vi "Z_state.vi"(9 "Alarm":bool[](array[boolean])=[FALSE, FALSE], 10 "Z_In":T4={"Z_Source"=enum."hand", "Z_Set_State"=enum."initialization", "ZM_State"=enum."initialization"}, 11 "Z_state in":refnum<class "valve_VCH_Z_state.lvclass">) -> (3 "Z_state out":refnum<class "valve_VCH_Z_state.lvclass">)   [LabVIEW 2019, in "valve_VCH_Z_state.lvclass"]
uses:
  valve_VCH_Z_state.lvclass
  D:/my_projects/projects/Algorithms/Labview/19/Sequence/State/State.lvclass
  Heating/ctl/Z_source.ctl
  ctl/Z_State_VCH.ctl
  ctl/ZM_State_VCH.ctl
  valve_VCH_Z_state.lvclass/valve_VCH_Z_state.ctl
  Sequence/State/State.lvclass
  Valves.lvlib
  Heating/Heating.lvlib
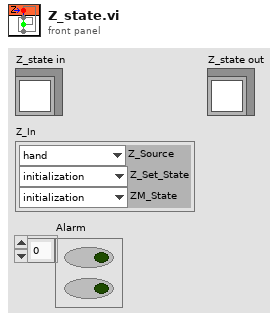
[diagram p1: front panel]
types:
  T1 = typedef "Heating.lvlib/Z_source.ctl" = enum8{"initialize", "local disabled", "local hand", "hand", "auto", "dist"}
  T2 = typedef "Valves.lvlib/Z_State_VCH.ctl" = enum8{"initialization", "alarm", "disabled", "not ready", "closed ready", "reserv", "reserv1", "reserv2", "reserv3", "check", "on min", "open", "on (closed)"}
  T3 = typedef "Valves.lvlib/ZM_State_VCH.ctl" = enum8{"initialization", "closed", "big_pause", "little_pause", "open", "close_cmd"}
  T4 = cluster{"Z_Source":T1, "Z_Set_State":T2, "ZM_State":T3}
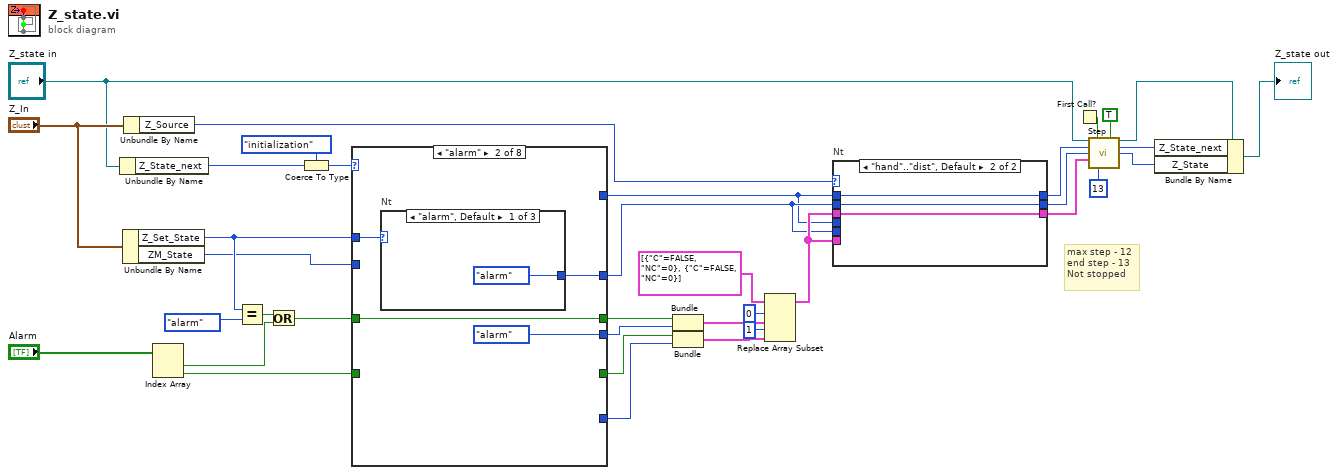
[diagram p0: block diagram]
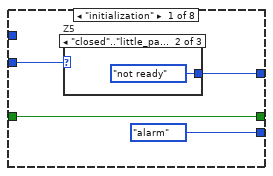
[diagram p2: hidden frame]
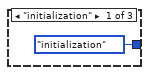
[diagram p3: hidden frame]
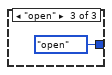
[diagram p4: hidden frame]
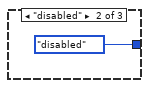
[diagram p5: hidden frame]
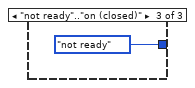
[diagram p6: hidden frame]
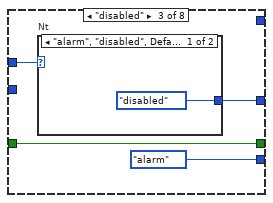
[diagram p7: hidden frame]
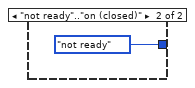
[diagram p8: hidden frame]
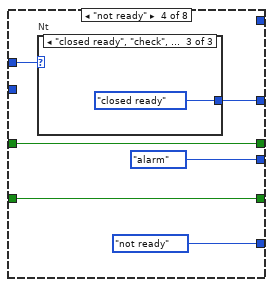
[diagram p9: hidden frame]
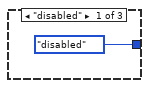
[diagram p10: hidden frame]
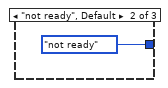
[diagram p11: hidden frame]
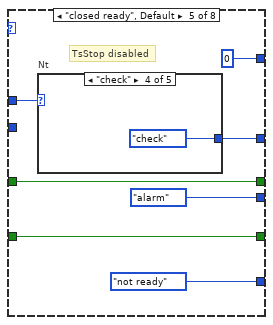
[diagram p12: hidden frame]
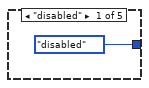
[diagram p13: hidden frame]
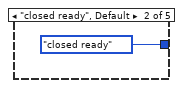
[diagram p14: hidden frame]
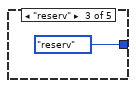
[diagram p15: hidden frame]
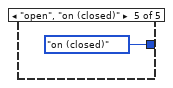
[diagram p16: hidden frame]
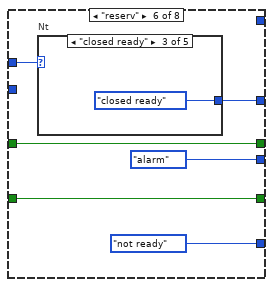
[diagram p17: hidden frame]
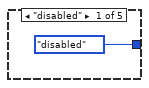
[diagram p18: hidden frame]
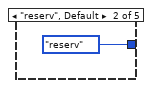
[diagram p19: hidden frame]
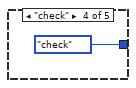
[diagram p20: hidden frame]
diagram:
  # "max step - 12\nend step - 13\nNot stopped"
  n1 = Unbundle By Name("Z_state in") -> ("Z_State_next"=w12:T2)
  n2 = Unbundle By Name("Z_In") -> ("Z_Set_State"=w8:T2, "ZM_State"=w7:T3)
  n3 = Unbundle By Name("Z_In") -> ("Z_Source"=w5:T1)
  n4 = Index Array(array="Alarm") -> (element #1=w16:bool, element #2=w15:bool)  [unwired: 2 in]
  n5 = Equal?(x=w8, y=Z_State_VCH."alarm" ("Z_State")) -> (x = y?=w32:bool)
  n6 = Or(x=w32, y=w16) -> (x .or. y?=w31:bool)
  n7 = Coerce To Type(0:w12, 1:Z_State_VCH."initialization" ("X5(DistSetSate) 2")) -> (2:w29:T2)
  n8 = case shown="\"alarm\"" w29 {
    tunnel: w31 -> [w40 w47 w54 w59 w72 w83 w96 w123]
    tunnel: w15 -> [_ _ _ w58 w68 w79 w92 w118]
    tunnel: w7 -> [w37 _ _ _ _ _ w91 w119]
    tunnel: [w40 w47 w54 w59 w72 w83 w96 w123] -> w23
    tunnel: [Z_State_VCH."alarm" ("state next") Z_State_VCH."alarm" ("state next") Z_State_VCH."alarm" ("state next") Z_State_VCH."alarm" ("state next") Z_State_VCH."alarm" ("state next") Z_State_VCH."alarm" ("state next") Z_State_VCH."alarm" ("state next") Z_State_VCH."alarm" ("state next")] -> w22
    tunnel: [w38 w46 w53 w61 w70 w81 w94 w121] -> w14
    tunnel: [_ _ _ Z_State_VCH."not ready" ("state next") Z_State_VCH."not ready" ("state next") Z_State_VCH."not ready" ("state next") w89 Z_State_VCH."not ready" ("state next")] -> w20
    tunnel: [_ _ _ w58 w68 w79 w90 w118] -> w21
    tunnel: [_ _ _ _ u32 0 ("pump param") _ _ _] -> w13
    tunnel: w8 -> [_ w45 w52 w62 w71 w82 w95 w122]
    frame "initialization" {
      n9 = case "Z5" shown="\"closed\"..\"little_pause\", Default" w37 {
        tunnel: [Z_State_VCH."initialization" ("state next") Z_State_VCH."not ready" ("state next") Z_State_VCH."open" ("state next")] -> w38
        frame "initialization" {
        }
        frame "closed".."little_pause", Default {
        }
        frame "open" {
        }
      }
    }
    frame "alarm" {
      n10 = case "Nt" shown="\"alarm\", Default" w45 {
        tunnel: [Z_State_VCH."alarm" ("state next") Z_State_VCH."disabled" ("state next") Z_State_VCH."not ready" ("state next")] -> w46
        frame "alarm", Default {
        }
        frame "disabled" {
        }
        frame "not ready".."on (closed)" {
        }
      }
    }
    frame "disabled" {
      n11 = case "Nt" shown="\"alarm\", \"disabled\", Default" w52 {
        tunnel: [Z_State_VCH."disabled" ("state next") Z_State_VCH."not ready" ("state next")] -> w53
        frame "alarm", "disabled", Default {
        }
        frame "not ready".."on (closed)" {
        }
      }
    }
    frame "not ready" {
      n12 = case "Nt" shown="\"closed ready\", \"check\", \"open\", \"on (closed)\"" w62 {
        tunnel: [Z_State_VCH."disabled" ("state next") Z_State_VCH."not ready" ("state next") Z_State_VCH."closed ready" ("state next")] -> w61
        frame "disabled" {
        }
        frame "not ready", Default {
        }
        frame "closed ready", "check", "open", "on (closed)" {
        }
      }
    }
    frame "closed ready", Default {
      # "TsStop disabled"
      n13 = case "Nt" shown="\"check\"" w71 {
        tunnel: [Z_State_VCH."disabled" ("state next") Z_State_VCH."closed ready" ("state next") Z_State_VCH."reserv" ("state next") Z_State_VCH."check" ("state next") Z_State_VCH."on (closed)" ("state next")] -> w70
        frame "disabled" {
        }
        frame "closed ready", Default {
        }
        frame "reserv" {
        }
        frame "check" {
        }
        frame "open", "on (closed)" {
        }
      }
    }
    frame "reserv" {
      n14 = case "Nt" shown="\"closed ready\"" w82 {
        tunnel: [Z_State_VCH."disabled" ("state next") Z_State_VCH."reserv" ("state next") Z_State_VCH."closed ready" ("state next") Z_State_VCH."check" ("state next") Z_State_VCH."open" ("state next")] -> w81
        frame "disabled" {
        }
        frame "reserv", Default {
        }
        frame "closed ready" {
        }
        frame "check" {
        }
        frame "open", "on (closed)" {
        }
      }
    }
    frame "check" {
      n15 = case "Nt" shown="\"disabled\"" w95 {
        tunnel: [w104 w108 Z_State_VCH."check" ("state next") w113] -> w94
        tunnel: w91 -> [w105 w109 _ w114]
        frame "disabled" {
          n16 = case "Z5" shown="\"open\"" w105 {
            tunnel: [Z_State_VCH."disabled" ("state next") Z_State_VCH."check" ("state next")] -> w104
            frame "closed".."little_pause", "close_cmd", Default {
            }
            frame "open" {
            }
          }
        }
        frame "closed ready", "reserv", Default {
          n17 = case "Z5" shown="\"closed\"..\"little_pause\", \"close_cmd\", Default" w109 {
            tunnel: [Z_State_VCH."closed ready" ("state next") Z_State_VCH."check" ("state next")] -> w108
            frame "closed".."little_pause", "close_cmd", Default {
            }
            frame "open" {
            }
          }
        }
        frame "check" {
        }
        frame "open", "on (closed)" {
          n18 = case "Z5" shown="\"closed\"..\"little_pause\", \"close_cmd\", Default" w114 {
            tunnel: [Z_State_VCH."on (closed)" ("state next") Z_State_VCH."open" ("state next")] -> w113
            frame "closed".."little_pause", "close_cmd", Default {
            }
            frame "open" {
            }
          }
        }
      }
      n19 = case "Nt" shown="True" w92 {
        selector: w92 -> [w97 w102]
        tunnel: [w98 Z_State_VCH."check" ("state next")] -> w89
        tunnel: w91 -> [w99 _]
        tunnel: [w97 w102] -> w90
        frame True {
          n20 = case "Z5" shown="\"closed\"..\"little_pause\", \"close_cmd\", Default" w99 {
            tunnel: [Z_State_VCH."not ready" ("state next") Z_State_VCH."check" ("state next")] -> w98
            frame "closed".."little_pause", "close_cmd", Default {
            }
            frame "open" {
            }
          }
        }
        frame False {
        }
      }
    }
    frame "open", "on (closed)" {
      n21 = case "Nt" shown="\"open\", \"on (closed)\"" w122 {
        tunnel: [w124 w128 w132] -> w121
        tunnel: w119 -> [w125 w129 w133]
        frame "disabled" {
          n22 = case "Z5" shown="\"open\"" w125 {
            tunnel: [Z_State_VCH."disabled" ("state next") Z_State_VCH."open" ("state next")] -> w124
            frame "closed".."little_pause", "close_cmd", Default {
            }
            frame "open" {
            }
          }
        }
        frame "closed ready", "reserv", Default {
          n23 = case "Z5" shown="\"closed\"..\"little_pause\", \"close_cmd\", Default" w129 {
            tunnel: [Z_State_VCH."closed ready" ("state next") Z_State_VCH."open" ("state next")] -> w128
            frame "closed".."little_pause", "close_cmd", Default {
            }
            frame "open" {
            }
          }
        }
        frame "open", "on (closed)" {
          n24 = case "Z5" shown="\"open\"" w133 {
            tunnel: [Z_State_VCH."on (closed)" ("state next") Z_State_VCH."open" ("state next")] -> w132
            frame "closed".."little_pause", "close_cmd", Default {
            }
            frame "open" {
            }
          }
        }
      }
    }
  }
  n25 = Bundle(w23, "state next"=w22) -> (w26:cluster{bool, "state next":T2})  [unwired: 1 in]
  n26 = Bundle("Alarm"=w21, "state next"=w20) -> (w24:cluster{"Alarm":bool, "state next":T2})  [unwired: 1 in]
  n27 = Replace Array Subset(array=cluster{"C":bool, "NC":u32}[] [{"C"=FALSE, "NC"=0}, {"C"=FALSE, "NC"=0}] ("appended array"), new element #1=w26, index #1=0 ("index"), new element #2=w24, index #2=1 ("index")) -> (w18:cluster{"C":bool, "NC":u32}[])
  n28 = case "Nt" shown="\"hand\"..\"dist\", Default" w5 {
    tunnel: w14 -> [_ w141]
    tunnel: w18 -> [_ w140]
    tunnel: [w137 w141] -> w10
    tunnel: [w138 w140] -> w11
    tunnel: w14 -> [w137 _]
    tunnel: w18 -> [w138 _]
    tunnel: w13 -> [_ w139]
    tunnel: [w136 w139] -> w9
    tunnel: w13 -> [w136 _]
    frame "local disabled", "local hand" {
    }
    frame "hand".."dist", Default {
    }
  }
  n29 = First Call?() -> (First Call?: T/F=w36:bool)
  n30 = call "Step.vi"("State in"="Z_state in", "Reset"=w36, "Start in"=TRUE ("Start"), "t"=w9, "Nt"=w10, "C_table"=w11, "N end step"=u32 13) -> ("State out"=w1:refnum<class "valve_VCH_Z_state.lvclass">, "N next"=w33:u32, "N curr"=w34:u32)  [unwired: 5 in, 1 out]
  n31 = Bundle By Name(cluster=w1, "Z_State_next"=w33, "Z_State"=w34) -> (→"Z_state out":refnum<class "valve_VCH_Z_state.lvclass">)
